vi "Laboratory_practice9.vi"() -> ()   [LabVIEW 2022 SP3]
uses:
  <vilib>/Analysis/3filter.llb/Filter Passband Type.ctl
  <vilib>/Analysis/3filter.llb/Butterworth Filter (DBL).vi
  <vilib>/Analysis/NI_AALBase.lvlib
panel:
  in  "stop":bool
  out "RMS":dbl
  out "Waveform Graph":dynamicdata(graph)
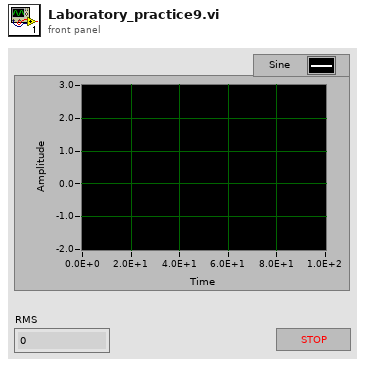
[diagram p1: front panel]
types:
  T1 = typedef "NI_AALBase.lvlib/Filter Passband Type.ctl" = enum32{"Lowpass", "Highpass", "Bandpass", "Bandstop"}
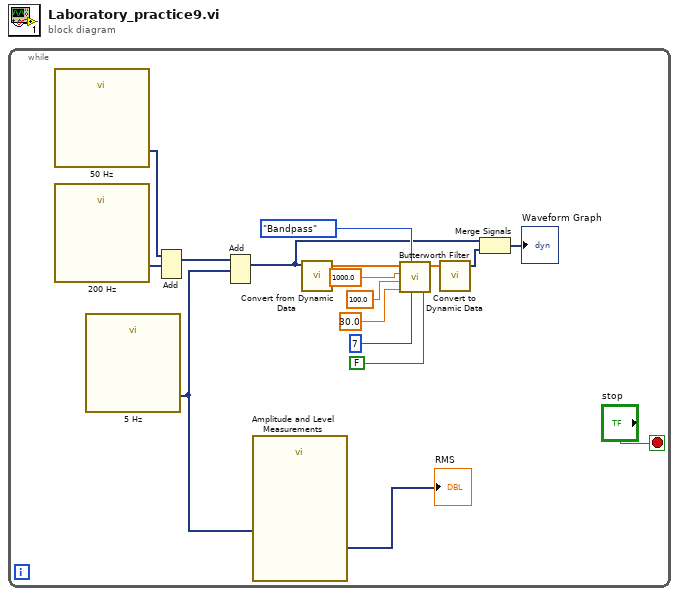
[diagram p0: block diagram]
diagram:
  n1 = while {
    stop <- "stop" stop-if-true
    n2 = call "50 Hz"() -> ("Sine"=w15:dynamicdata)  [unwired: 14 in, 1 out]
    n3 = call "200 Hz"() -> ("Sine"=w13:dynamicdata)  [unwired: 14 in, 1 out]
    n4 = call "5 Hz"() -> ("Sine"=w12:dynamicdata)  [unwired: 14 in, 1 out]
    n5 = Add(1:w13, 2:w15) -> (0:w14:dynamicdata)  [unwired: 1 in, 1 out]
    n6 = Add(1:w12, 2:w14) -> (0:w2:dynamicdata)  [unwired: 1 in, 1 out]
    n7 = call "Amplitude and Level Measurements"("Signals"=w12) -> ("RMS"=→"RMS":dynamicdata)  [unwired: 12 in, 2 out]
    n8 = call "Convert from Dynamic Data"("Dynamic Data Type"=w2) -> ("Array"=w1:dbl[])  [unwired: 3 in]
    n9 = call-poly <vilib>:"Butterworth Filter.vi"("init/cont (init:F)"=FALSE, "order"=7, "filter type"=Filter_Passband_Type."Bandpass", "low cutoff freq: fl"=30.0, "high cutoff freq: fh"=100.0, "sampling freq: fs"=1000.0, "X"=w1) -> ("Filtered X"=w10:dbl[])  [unwired: 1 in, 1 out]
    n10 = call "Convert to Dynamic Data"("Array"=w10) -> ("Dynamic Data Type"=w9:dynamicdata)  [unwired: 3 in]
    n11 = Merge Signals(w2, w9) -> (→"Waveform Graph":dynamicdata)
  }
